vi "Read subject.vi"(8 "error in (no error)":errorcluster, 11 "OperationLogger (proxy) in":refnum<class "OperationLogger (proxy).lvclass">) -> (0 "error out":errorcluster, 2 "Normal Proxy.lvlib:Subject.lvclass":refnum<class "Subject.lvclass">, 3 "OperationLogger (proxy) out":refnum<class "OperationLogger (proxy).lvclass">)   [LabVIEW 2014, in "forcible Proxy.lvlib" / "OperationLogger (proxy).lvclass"]
uses:
  OperationLogger (proxy).lvclass
  Subject/Subject.lvclass
  OperationLogger (proxy).lvclass/OperationLogger (proxy).ctl
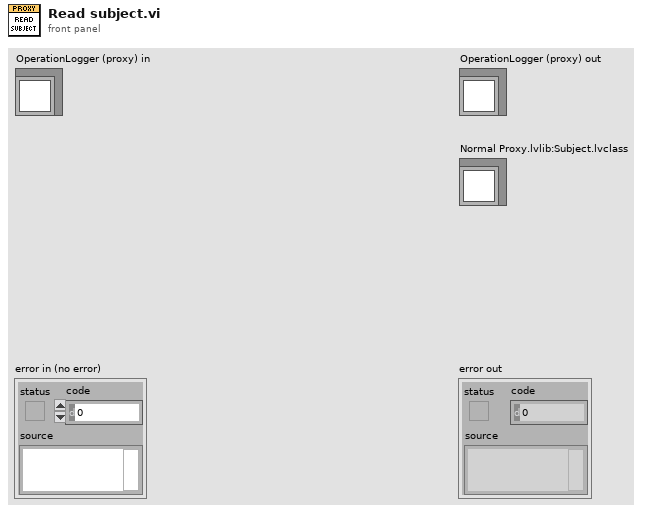
[diagram p1: front panel]
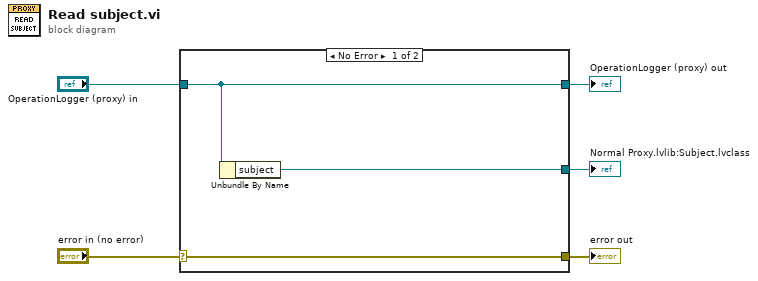
[diagram p0: block diagram]
diagram:
  n1 = case shown="No Error" "error in (no error)" {
    selector: "error in (no error)" -> [w8 w9]
    tunnel: [w8 w9] -> w4
    tunnel: [w7 w10] -> w2
    tunnel: "OperationLogger (proxy) in" -> [w7 w10]
    tunnel: [w6 _] -> w1
    frame No Error {
      n2 = Unbundle By Name(w7) -> ("subject"=w6:refnum<class "Subject.lvclass">)
    }
    frame Error {
    }
  }
  "error out" <- w4
  "OperationLogger (proxy) out" <- w2
  "Normal Proxy.lvlib:Subject.lvclass" <- w1
